vi "GUI Get Paths.vi"(11 "error in (no error)":errorcluster) -> (4 "Paths":T1, 15 "error out":errorcluster)   [LabVIEW 2019]
uses:
  TypeDef/GUI Paths.ctl
  <vilib>/Utility/sysdir.llb/System Directory Type.ctl
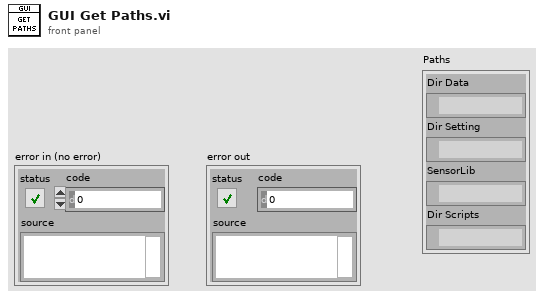
[diagram p1: front panel]
types:
  T1 = typedef "GUI Paths.ctl" = cluster{"Dir Data":path, "Dir Setting":path, "SensorLib":path, "Dir Scripts":path}
  T2 = typedef "System Directory Type.ctl" = i32
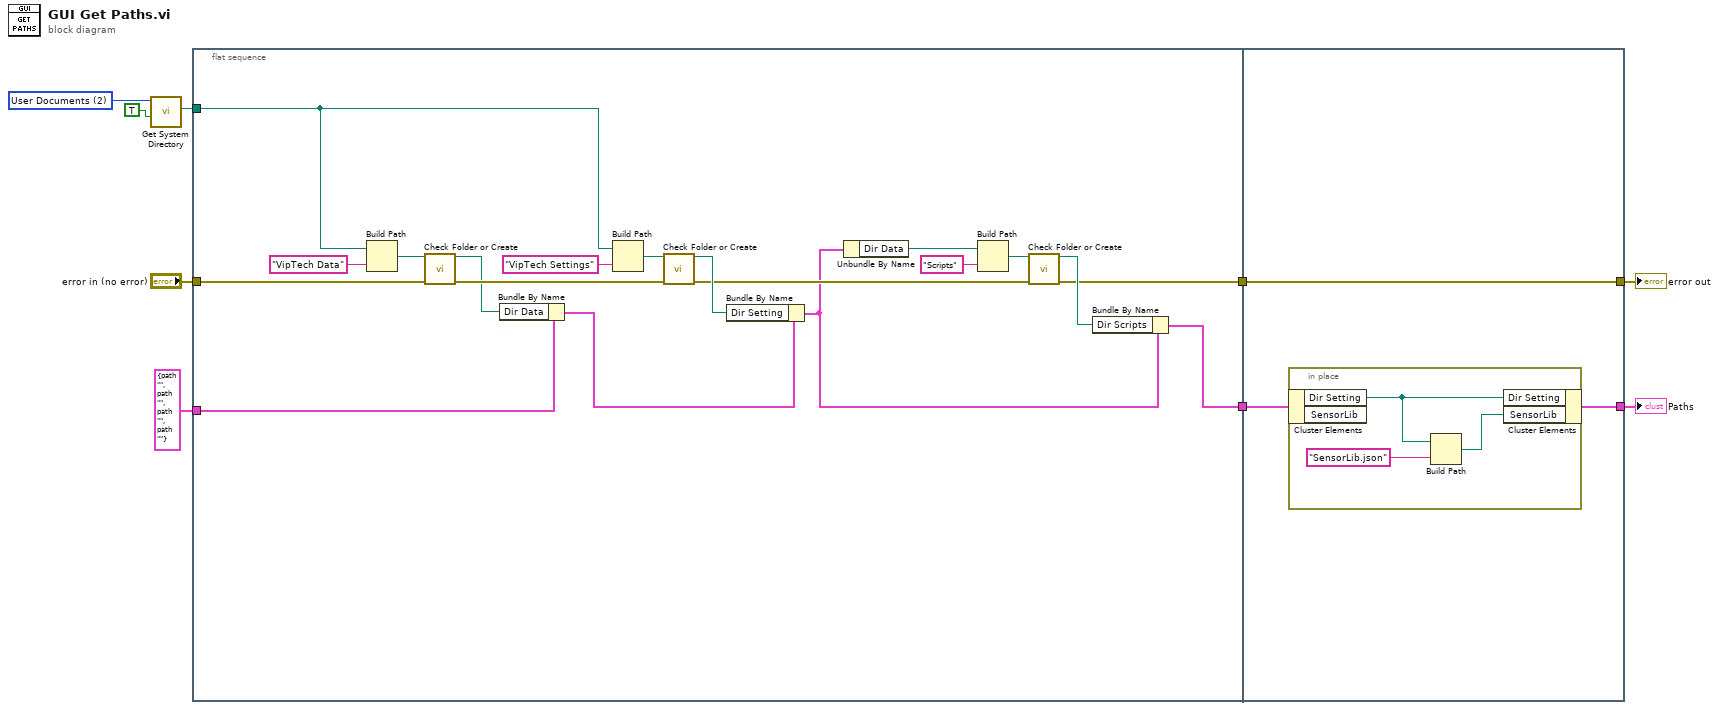
[diagram p0: block diagram]
diagram:
  w5 = T2 2 items=["User Home"=0, "User Desktop"=1, "User Documents"=2, "User Application Data"=3, "User Preferences"=4, "User Temporary"=5, "Public Documents"=6, "Public Application Data"=7, "Public Preferences"=8, "Public Cache"=13, "System Core Libraries"=9, "System Installed Libraries"=10, "Application Files"=11, "Boot Volume Root"=12] ("system directory type")
  n1 = call <vilib>:"Get System Directory.vi"("create directory if not found? (F)"=TRUE, "system directory type"=w5) -> ("system directory"=w4:path)  [unwired: 9 in]
  n2 = flat-sequence {
    tunnel: "error in (no error)" -> [w23]
    tunnel: T1 {"Dir Data"=path "", "Dir Setting"=path "", "SensorLib"=path "", "Dir Scripts"=path ""} ("Paths") -> [w22]
    tunnel: w4 -> [w19]
    tunnel: [w15] -> w3
    tunnel: [w13] -> w1
    tunnel: [w30] -> w7
    tunnel: w3 -> [w31]
    tunnel: [w29] -> w2
    tunnel: w1 -> [w29]
    frame #0 {
      n3 = Build Path(base path=w19, name or relative path="VipTech Data") -> (appended path=w25:path)
      n4 = call "Check Folder or Create.vi"("path"=w25, "error in (no error)"=w23) -> ("dup path"=w12:path, "error out"=w24:errorcluster)  [unwired: 12 in]
      n5 = Bundle By Name(cluster=w22, "Dir Data"=w12) -> (w21:T1)
      n6 = Build Path(base path=w19, name or relative path="VipTech Settings") -> (appended path=w26:path)
      n7 = call "Check Folder or Create.vi"("path"=w26, "error in (no error)"=w24) -> ("dup path"=w20:path, "error out"=w14:errorcluster)  [unwired: 12 in]
      n8 = Bundle By Name(cluster=w21, "Dir Setting"=w20) -> (w11:T1)
      n9 = Unbundle By Name(w11) -> ("Dir Data"=w10:path)
      n10 = Build Path(base path=w10, name or relative path="Scripts") -> (appended path=w17:path)
      n11 = call "Check Folder or Create.vi"("path"=w17, "error in (no error)"=w14) -> ("dup path"=w18:path, "error out"=w13:errorcluster)  [unwired: 12 in]
      n12 = Bundle By Name(cluster=w11, "Dir Scripts"=w18) -> (w15:T1)
    }
    frame #1 {
      n13 = in-place {
        n14 = in-place-cluster #1(w31) -> ("Dir Setting"=w34:path)  [unwired: 1 out]
        n15 = Build Path(base path=w34, name or relative path="SensorLib.json") -> (appended path=w32:path)
        n16 = in-place-cluster #1("Dir Setting"=w34, "SensorLib"=w32) -> (w30:T1)
      }
    }
  }
  "error out" <- w2
  "Paths" <- w7
